vi "PID.vi"   [LabVIEW 2016, in "Moving Motor.lvrbt"]
uses:
  Moving Motor.lvrbt
  <vilib>/NXT/Block Support/NXT_InputPort.ctl
  <vilib>/NXT/Hardware/Plugins/Tetrix DC Motor/TetrixDCMotorAddress.ctl
  <vilib>/NXT/Dual Mode Library/Sensors/EV3_Color_Reflect.vi
  <vilib>/NXT/NXTIO Xnodes/NXTIONodeSubVIs/TETRIX IO Move DC Motors.vi
  <vilib>/NXT/NXTIO Xnodes/AddressXNode/NXTIOAddress.xnode
  <vilib>/NXT/NXTIO Xnodes/NXTIOXNode/NXTIO.xnode
  <vilib>/NXT/Subs/LVHSConnector.ctl
  <vilib>/NXT/LegoClasses/BrickReference/BrickReference.lvclass
types:
  T1 = typedef "NXT_InputPort.ctl" = u32
  T2 = typedef "LVHSConnector.ctl" = refnum<class "BrickReference.lvclass">
  T3 = typedef "TetrixDCMotorAddress.ctl" = i32
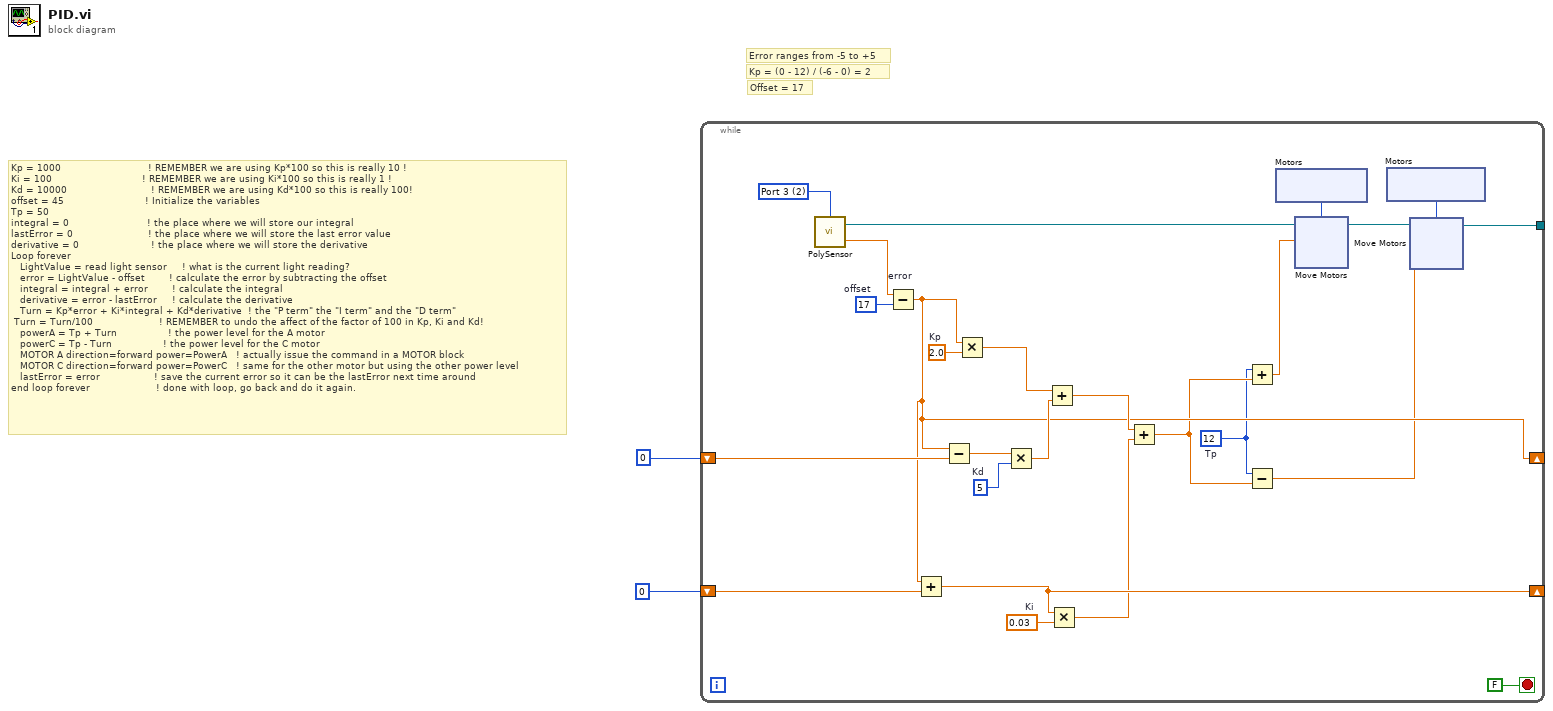
[diagram p0: block diagram]
diagram:
  # "Kp = 1000                             ! REMEMBER we are using Kp*100 so this is really 10 !\nKi = 100                              ! REMEMBER we are using Ki*100 so this is really 1 !\nKd = 10000                            ! REMEMBER we are using Kd*100 so this is really 100!\noffset = 45                           ! Initialize the variables\nTp = 50 \nintegral = 0                          ! the place where we will store our integral\nlastError = 0                         ! the place where we will store the last error value\nderivative = 0                        ! the place where we will store the derivative\nLoop forever\n   LightValue = read light sensor     ! what is the current light reading?\n   error = LightValue - offset        ! calculate the error by subtracting the offset\n   integral = integral + error        ! calculate the integral \n   derivative = error - lastError     ! calculate the derivative\n   Turn = Kp*error + Ki*integral + Kd*derivative  ! the \"P term\" the \"I term\" and the \"D term\"\n Turn = Turn/100                      ! REMEMBER to undo the affect of the factor of 100 in Kp, Ki and Kd!\n   powerA = Tp + Turn                 ! the power level for the A motor\n   powerC = Tp - Turn                 ! the power level for the C motor\n   MOTOR A direction=forward power=PowerA   ! actually issue the command in a MOTOR block\n   MOTOR C direction=forward power=PowerC   ! same for the other motor but using the other power level\n   lastError = error                  ! save the current error so it can be the lastError next time around\nend loop forever                      ! done with loop, go back and do it again."
  # "Offset = 17"
  # "Kp = (0 - 12) / (-6 - 0) = 2"
  # "Error ranges from -5 to +5"
  n1 = while {
    tunnel: [w21] -> _
    shift-right: [w7] -> _
    shift-left: 0 -> [w16]
    shift-right: [w11] -> _
    shift-left: 0 -> [w13]
    stop <- FALSE stop-if-true
    w5 = 12  # Tp
    w12 = 0.03  # Ki
    w14 = 5  # Kd
    w18 = 2.0  # Kp
    w19 = i16 17  # offset
    w26 = T1 2 items=["Port 1"=0, "Port 2"=1, "Port 3"=2, "Port 4"=3, "MidColor"=5] ("Port (Port 3)")
    n2 = call-poly <vilib>:"PolySensor.vi"("Port (Port 1)"=w26) -> ("Scaled Value"=w20:sgl, "NXT/EV3"=w23:T2)  [unwired: 2 in]
    n3 = Subtract "error"(x=w20, y=w19) -> (x-y=w7:sgl)
    n4 = Add(x=w7, y=w13) -> (x+y=w11:sgl)
    n5 = Subtract(x=w7, y=w16) -> (x-y=w15:sgl)
    n6 = Multiply(x=w7, y=w18) -> (x*y=w17:dbl)
    n7 = Multiply(x=w15, y=w14) -> (x*y=w10:sgl)
    n8 = Add(x=w17, y=w10) -> (x+y=w9:dbl)
    n9 = Multiply(x=w11, y=w12) -> (x*y=w8:dbl)
    n10 = Add(x=w9, y=w8) -> (x+y=w6:dbl)
    n11 = Add(x=w5, y=w6) -> (x+y=w4:dbl)
    n12 = Subtract(x=w5, y=w6) -> (x-y=w3:dbl)
    n13 = xnode "Motors"() -> ("Motor"=w25:T3)
    n14 = xnode "Move Motors"("Power/Speed 1"=w4, "Motors"=w25, "NXT/EV3"=w23) -> ("NXT/EV3"=w22:T2)
    n15 = xnode "Motors"() -> ("Motor"=w24:T3)
    n16 = xnode "Move Motors"("Power/Speed 1"=w3, "Motors"=w24, "NXT/EV3"=w22) -> ("NXT/EV3"=w21:T2)
  }
